vi "ccidinfo-r.vi"(1 "Data Type":T1, 2 "Slot":T2) -> (0 "Data":string)   [LabVIEW 2013]
uses:
  SystemCode/SysControl/Slot.ctl
  PDINFO.ctl
  GlobalValue.vi
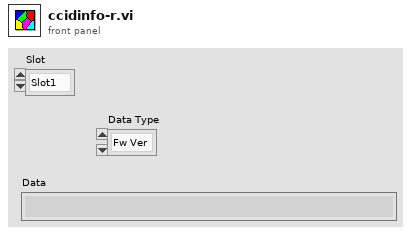
[diagram p1: front panel]
types:
  T1 = typedef "PDINFO.ctl" = enum16{"Fw Ver", "HW Ver", "CCID", "WiFiName", "DevID", "SN", "TUID", "CertifID", "PdTime", "Provider", "WiFiPassword", "Imei", "AuthCode", "Reserved1", "Reserved2", "Reserved3"}
  T2 = typedef "Slot.ctl" = enum16{"Slot1", "Slot2", "Slot3", "Slot4"}
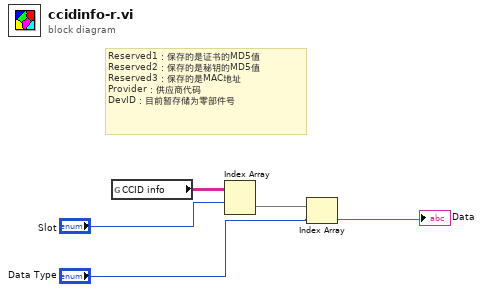
[diagram p0: block diagram]
diagram:
  # "Reserved1：保存的是证书的MD5值\nReserved2：保存的是秘钥的MD5值\nReserved3：保存的是MAC地址\nProvider：供应商代码\nDevID：目前暂存储为零部件号"
  n1 = global read "GlobalValue.vi" "CCID info"() -> (w5:string[][])
  n2 = Index Array(array=w5, index (row)="Slot") -> (element=w3:string[])  [unwired: 1 in]
  n3 = Index Array(array=w3, index="Data Type") -> (element=→"Data":string)
